vi "Timed Write to Hardware.vi"(8 "error in":errorcluster, 9 "trigger values":dbl[](array[numeric]), 10 "values in":dbl[](array[numeric]), 11 "execution unit":refnum<class "Execution Unit.lvclass">) -> (0 "error out":errorcluster, 1 "trigger values out":dbl[](array[numeric]), 2 "values out":dbl[](array[numeric]), 3 "execution unit out":refnum<class "Execution Unit.lvclass">)   [LabVIEW 2020, in "AIM MIL-STD-1553 Engine.lvlib" / "Custom Device.lvlib"]
uses:
  Custom Device.lvlib
  Interfaces/Execution Unit/Execution Unit.lvclass
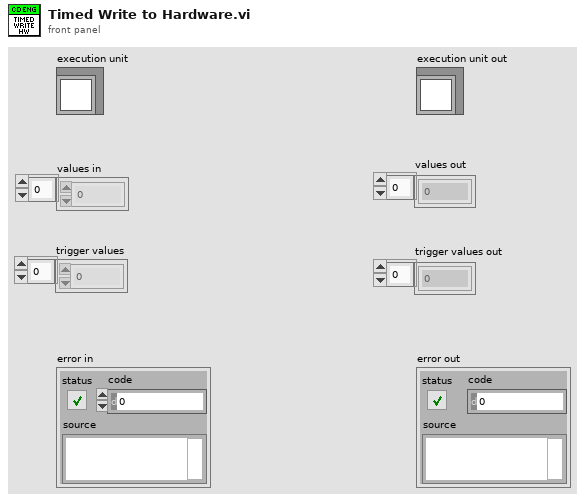
[diagram p1: front panel]
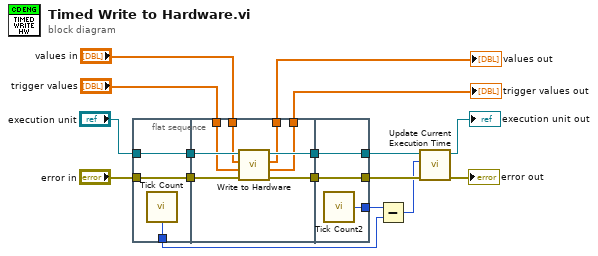
[diagram p0: block diagram]
diagram:
  n1 = flat-sequence {
    tunnel: "error in" -> [w19]
    tunnel: "execution unit" -> [w20]
    tunnel: [w20] -> w17
    tunnel: [w19] -> w16
    tunnel: [w18] -> w13
    tunnel: w17 -> [w28]
    tunnel: w16 -> [w27]
    tunnel: [w26] -> w15
    tunnel: [w25] -> w14
    tunnel: [w24] -> w10
    tunnel: [w23] -> w9
    tunnel: "values in" -> [w22]
    tunnel: "trigger values" -> [w21]
    tunnel: [w30] -> w6
    tunnel: [w31] -> w5
    tunnel: w15 -> [w31]
    tunnel: w14 -> [w30]
    tunnel: [w29] -> w12
    frame #0 {
      n2 = call "Tick Count"() -> ("Tick Count(uSec)"=w18:u32)
    }
    frame #1 {
      n3 = call-dynamic "Write to Hardware.vi"("error in (no error)"=w27, "Trigger Values"=w21, "Values in"=w22, "Execution Unit in"=w28) -> ("error out"=w25:errorcluster, "Trigger Values out"=w23:dbl[], "Values out"=w24:dbl[], "Execution Unit out"=w26:refnum<class "Execution Unit.lvclass">)  [unwired: 4 in]
    }
    frame #2 {
      n4 = call "Tick Count2"() -> ("Tick Count(uSec)"=w29:u32)
    }
  }
  n5 = Subtract(x=w12, y=w13) -> (x-y=w3:u32)
  n6 = call-dynamic "Update Current Execution Time.vi"("error in (no error)"=w6, "Current Execution Time (us)"=w3, "Execution Unit in"=w5) -> ("error out"=→"error out":errorcluster, "Execution Unit out"=→"execution unit out":refnum<class "Execution Unit.lvclass">)  [unwired: 7 in]
  "values out" <- w10
  "trigger values out" <- w9
